vi "Autonomous Independent.vi"   [LabVIEW 2015]
doc: "This VI is called when autonomous begins, and will automatically be terminated when autonomous ends. You can carry out timed or sensor driven robot movement independently without needing to return to the caller."
uses:
  <vilib>/Rock Robotics/WPI/Utilities/WPI_GetSetVariantRefNum.vi
  <vilib>/Rock Robotics/Network Tables/NT Read Number.vi
  Robot Global Data.vi
  <vilib>/Rock Robotics/WPI/RobotDrive/WPI_RobotDriveMecanumDrive_Cartesian.vi
  <vilib>/Rock Robotics/Network Tables/NT Write Numeric Array.vi
panel:
  # "Be sure to right-click and choose Data Operations>>Make Current Value default if you want to save the array values with the VI"
types:
  T1 = typedef "WPI_JoystickDevRef.ctl" = cluster{"Device":T2}
  T2 = typedef "WPI_JoystickDeviceEnum.ctl" = enum16{"USB 0", "USB 1", "USB 2", "USB 3", "USB 4", "USB 5"}
  T3 = typedef "WPI_RobotDriveDevRef.ctl" = cluster{"DevStatus":errorcluster, "Motors[]":T4[], "Square Inputs":bool, "Max Output":dbl}
  T4 = typedef "WPI_MotorControlDeviceRef.ctl" = cluster{"DeviceStatus":errorcluster, "Type":T5, "PWM":cluster{"PWM Channel":T6, "DeadBand":T7}, "CAN":cluster{"Device Number":u8, "Control Mode":T8, "Semaphore":T9, "Max Vout":dbl, "TalonSRX Control Mode":T10}, "Invert":bool}
  T5 = typedef "WPI_MotorControlType.ctl" = enum16{"PWM", "CAN", "CANTalonSRX"}
  T6 = typedef "FPGA_DIOPWMChannel.ctl" = enum8{"PWM 0", "PWM 1", "PWM 2", "PWM 3", "PWM 4", "PWM 5", "PWM 6", "PWM 7", "PWM 8", "PWM 9", "PWM MXP 0", "PWM MXP 1", "PWM MXP 2", "PWM MXP 3", "PWM MXP 4", "PWM MXP 5", "PWM MXP 6", "PWM MXP 7", "PWM MXP 8", "PWM MXP 9", "Invalid"}
  T7 = typedef "WPI_PWMDeadband.ctl" = cluster{"Name":string, "maxPositivePwm":i32, "minPositivePwm":i32, "centerPwm":i32, "maxNegativePwm":i32, "minNegativePwm":i32, "angularRange":u16}
  T8 = typedef "WPI_CANJaguar_ControlMode.ctl" = enum8{"Percent VBus", "Current", "Speed", "Position", "Voltage"}
  T9 = typedef "Semaphore RefNum" = refnum<k1>
  T10 = typedef "WPI_CANTalonSRX_APIControlMode.ctl" = enum8{"Percent VBus", "Speed", "Position", "Slave", "Unchanged / Invalid", "Voltage Compensation", "Current", "Motion Profile"}
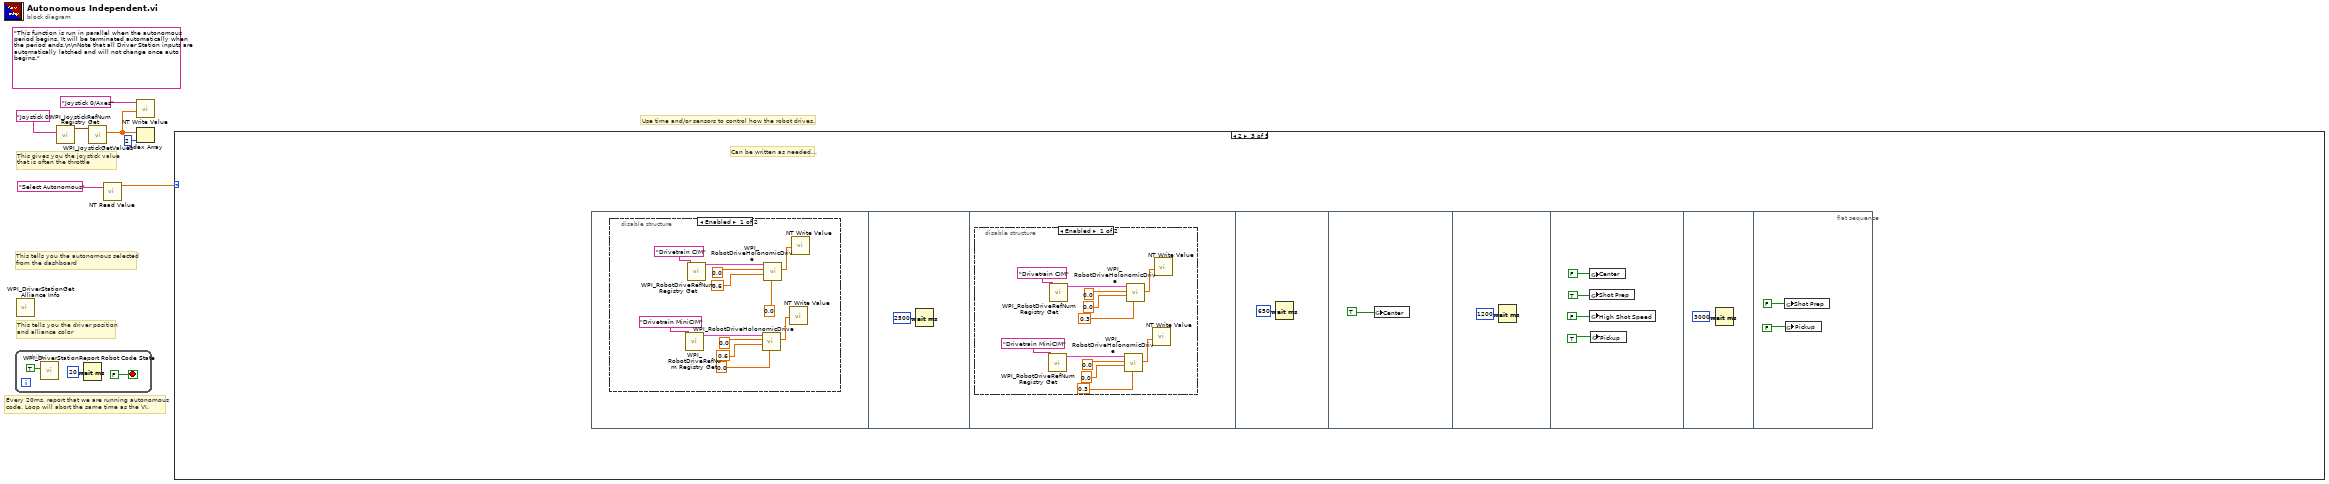
[diagram p0: block diagram]
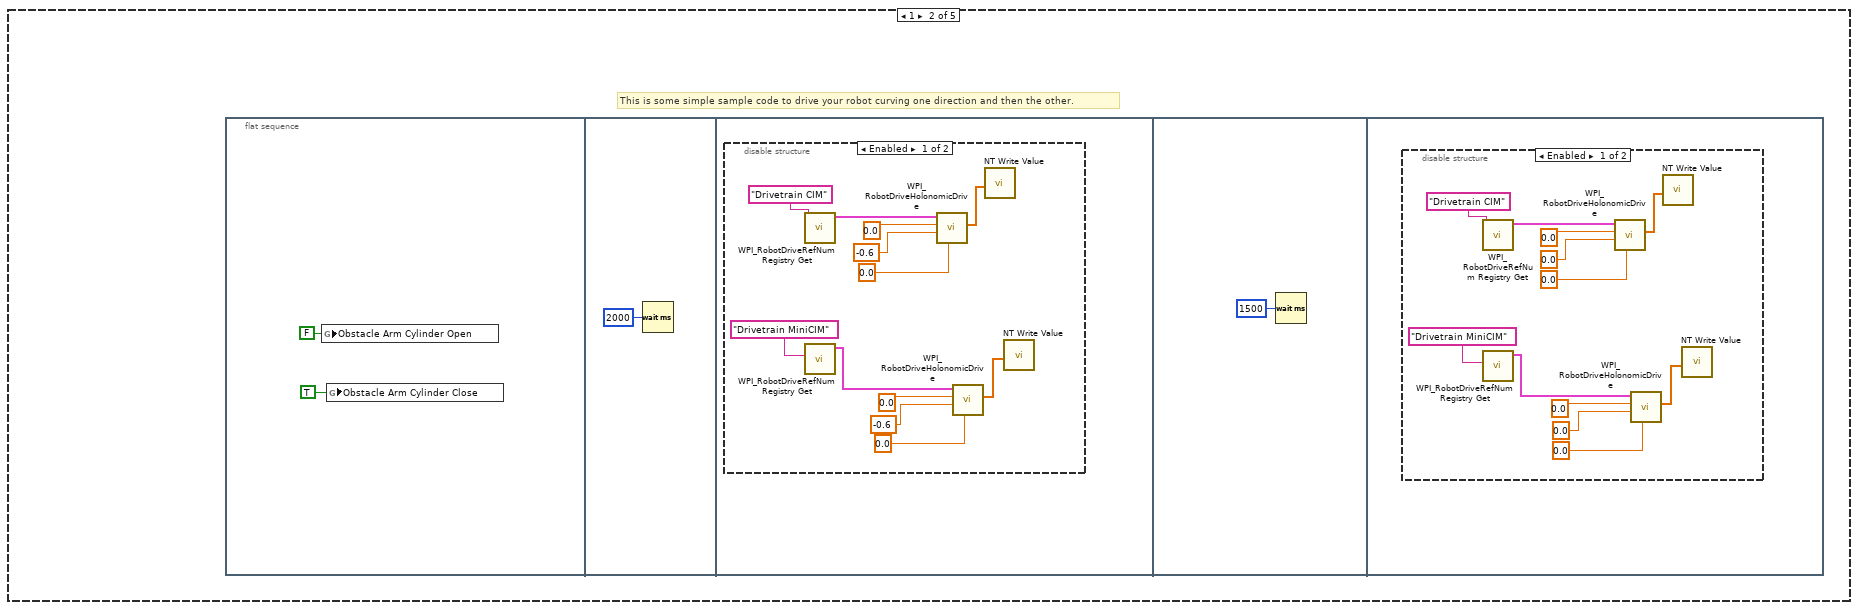
[diagram p3: hidden frame]
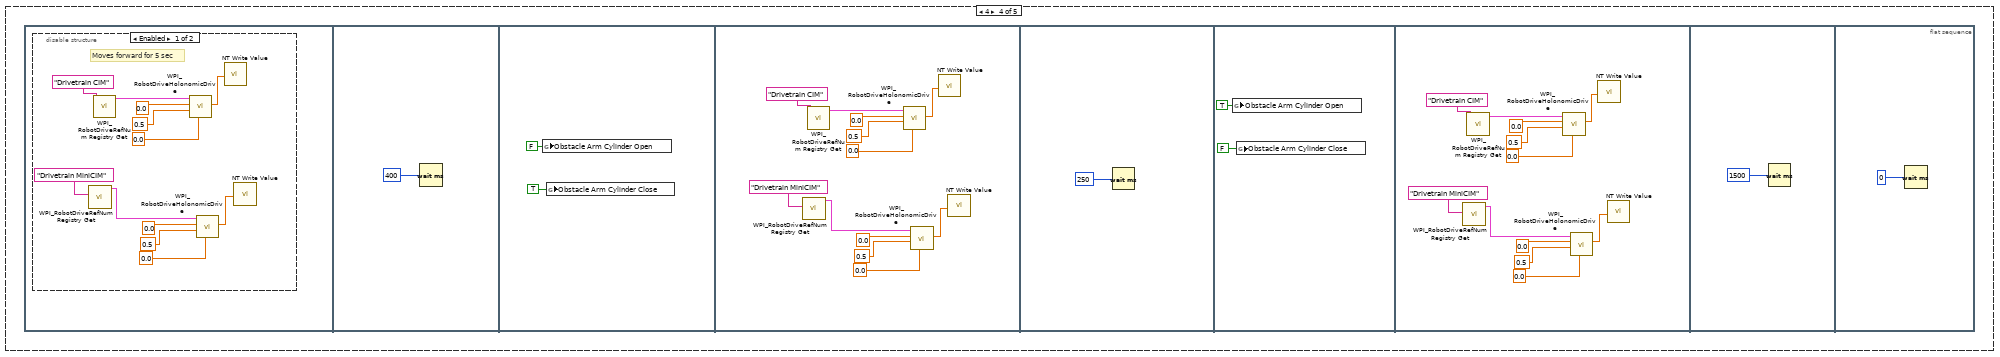
[diagram p8: hidden frame]
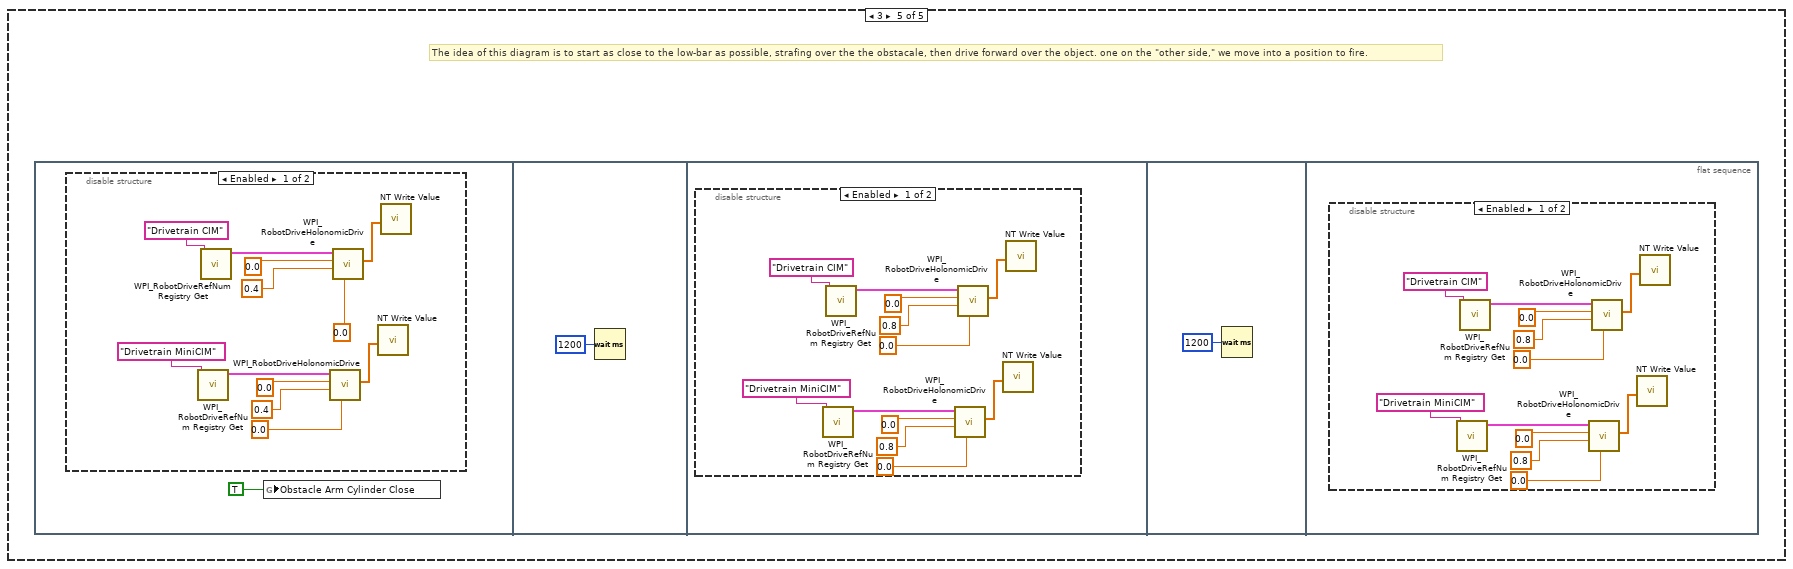
[diagram p10: hidden frame]
diagram:
  (unwired) "This function is run in parallel when the autonomous period begins. It will be terminated automatically when the period ends.\n\nNote that all Driver Station inputs are automatically latched and will not change once auto begins."
  # "This tells you the autonomous selected\nfrom the dashboard"
  # "Every 20ms, report that we are running autonomous\ncode. Loop will abort the same time as the VI."
  # "This gives you the joystick value\nthat is often the throttle"
  # "Use time and/or sensors to control how the robot drives."
  # "This tells you the driver position\nand alliance color"
  n1 = while {
    stop <- FALSE stop-if-true
    n2 = call <vilib>:"WPI_DriverStationReport Robot Code State.vi"("Autonomous"=TRUE) -> ()  [unwired: 10 in, 1 out]
    n3 = Wait (ms)(milliseconds to wait=u32 20) -> ()  [unwired: 1 out]
  }
  n4 = call <vilib>:"WPI_DriverStationGet Alliance Info.vi"() -> ()  [unwired: 12 out]
  n5 = call <vilib>:"WPI_JoystickRefNum Registry Get.vi"("refnum name"="Joystick 0") -> ("JoystickDevRef"=w6:T1)  [unwired: 1 in, 9 out]
  n6 = call <vilib>:"WPI_JoystickGetValues.vi"("JoystickDevRef"=w6) -> ("Axes"=w3:dbl[])  [unwired: 6 in, 4 out]
  n7 = call-poly <vilib>:"NT Read Value.vi"("Name"="Select Autonomous") -> ("Numeric"=w1:dbl)  [unwired: 9 in, 1 out]
  n8 = call-poly <vilib>:"NT Write Value.vi"("Numeric Array"=w3, "Name"="Joystick 0/Axes") -> ()  [unwired: 9 in, 1 out]
  n9 = Index Array(array=w3, index=2) -> ()  [unwired: 1 out]
  n10 = case shown="2" w1 {
    frame 0, Default {
    }
    frame 1 {
      # "This is some simple sample code to drive your robot curving one direction and then the other."
      n11 = flat-sequence {
        frame #0 {
          n12 = global write "Robot Global Data.vi" "Obstacle Arm Cylinder Open"(FALSE) -> ()
          n13 = global write "Robot Global Data.vi" "Obstacle Arm Cylinder Close"(TRUE) -> ()
        }
        frame #1 {
          n14 = Wait (ms)(milliseconds to wait=u32 2000) -> ()  [unwired: 1 out]
        }
        frame #2 {
          n15 = disable-structure shown="Enabled" {
            frame Enabled {
              n16 = call <vilib>:"WPI_RobotDriveRefNum Registry Get.vi"("refnum name"="Drivetrain CIM") -> ("RobotDriveDevRef"=w21:T3)  [unwired: 1 in, 9 out]
              n17 = call <vilib>:"WPI_RobotDriveRefNum Registry Get.vi"("refnum name"="Drivetrain MiniCIM") -> ("RobotDriveDevRef"=w15:T3)  [unwired: 1 in, 9 out]
              n18 = call-poly <vilib>:"WPI_RobotDriveHolonomicDrive.vi"("Rotation"=0.0, "Y"=-0.6 ("X axis value"), "X"=0.0 ("X axis value"), "RobotDriveDevRef"=w21) -> ("Motor Values"=w22:dbl[])  [unwired: 5 in, 2 out]
              n19 = call-poly <vilib>:"WPI_RobotDriveHolonomicDrive.vi"("Rotation"=0.0, "Y"=-0.6 ("X axis value"), "X"=0.0 ("X axis value"), "RobotDriveDevRef"=w15) -> ("Motor Values"=w17:dbl[])  [unwired: 5 in, 2 out]
              n20 = call-poly <vilib>:"NT Write Value.vi"("Numeric Array"=w22) -> ()  [unwired: 10 in, 1 out]
              n21 = call-poly <vilib>:"NT Write Value.vi"("Numeric Array"=w17) -> ()  [unwired: 10 in, 1 out]
            }
            frame Disabled {
            }
          }
        }
        frame #3 {
          n22 = Wait (ms)(milliseconds to wait=u32 1500) -> ()  [unwired: 1 out]
        }
        frame #4 {
          n23 = disable-structure shown="Enabled" {
            frame Enabled {
              n24 = call <vilib>:"WPI_RobotDriveRefNum Registry Get.vi"("refnum name"="Drivetrain CIM") -> ("RobotDriveDevRef"=w34:T3)  [unwired: 1 in, 9 out]
              n25 = call <vilib>:"WPI_RobotDriveRefNum Registry Get.vi"("refnum name"="Drivetrain MiniCIM") -> ("RobotDriveDevRef"=w28:T3)  [unwired: 1 in, 9 out]
              n26 = call-poly <vilib>:"WPI_RobotDriveHolonomicDrive.vi"("Rotation"=0.0, "Y"=0.0 ("X axis value"), "X"=0.0 ("X axis value"), "RobotDriveDevRef"=w34) -> ("Motor Values"=w35:dbl[])  [unwired: 5 in, 2 out]
              n27 = call-poly <vilib>:"WPI_RobotDriveHolonomicDrive.vi"("Rotation"=0.0, "Y"=0.0 ("X axis value"), "X"=0.0 ("X axis value"), "RobotDriveDevRef"=w28) -> ("Motor Values"=w30:dbl[])  [unwired: 5 in, 2 out]
              n28 = call-poly <vilib>:"NT Write Value.vi"("Numeric Array"=w35) -> ()  [unwired: 10 in, 1 out]
              n29 = call-poly <vilib>:"NT Write Value.vi"("Numeric Array"=w30) -> ()  [unwired: 10 in, 1 out]
            }
            frame Disabled {
            }
          }
        }
      }
    }
    frame 2 {
      # "Can be written as needed..."
      n30 = flat-sequence {
        frame #0 {
          n31 = disable-structure shown="Enabled" {
            frame Enabled {
              n32 = call <vilib>:"WPI_RobotDriveRefNum Registry Get.vi"("refnum name"="Drivetrain MiniCIM") -> ("RobotDriveDevRef"=w40:T3)  [unwired: 1 in, 9 out]
              n33 = call <vilib>:"WPI_RobotDriveRefNum Registry Get.vi"("refnum name"="Drivetrain CIM") -> ("RobotDriveDevRef"=w46:T3)  [unwired: 1 in, 9 out]
              n34 = call-poly <vilib>:"WPI_RobotDriveHolonomicDrive.vi"("Rotation"=0.0, "Y"=0.6 ("X axis value"), "X"=0.0 ("X axis value"), "RobotDriveDevRef"=w40) -> ("Motor Values"=w41:dbl[])  [unwired: 5 in, 2 out]
              n35 = call-poly <vilib>:"WPI_RobotDriveHolonomicDrive.vi"("Rotation"=0.0, "Y"=0.6 ("X axis value"), "X"=0.0 ("X axis value"), "RobotDriveDevRef"=w46) -> ("Motor Values"=w47:dbl[])  [unwired: 5 in, 2 out]
              n36 = call-poly <vilib>:"NT Write Value.vi"("Numeric Array"=w41) -> ()  [unwired: 10 in, 1 out]
              n37 = call-poly <vilib>:"NT Write Value.vi"("Numeric Array"=w47) -> ()  [unwired: 10 in, 1 out]
            }
            frame Disabled {
            }
          }
        }
        frame #1 {
          n38 = Wait (ms)(milliseconds to wait=u32 2500) -> ()  [unwired: 1 out]
        }
        frame #2 {
          n39 = disable-structure shown="Enabled" {
            frame Enabled {
              n40 = call <vilib>:"WPI_RobotDriveRefNum Registry Get.vi"("refnum name"="Drivetrain MiniCIM") -> ("RobotDriveDevRef"=w53:T3)  [unwired: 1 in, 9 out]
              n41 = call <vilib>:"WPI_RobotDriveRefNum Registry Get.vi"("refnum name"="Drivetrain CIM") -> ("RobotDriveDevRef"=w59:T3)  [unwired: 1 in, 9 out]
              n42 = call-poly <vilib>:"WPI_RobotDriveHolonomicDrive.vi"("Rotation"=0.3, "Y"=0.0 ("X axis value"), "X"=0.0 ("X axis value"), "RobotDriveDevRef"=w53) -> ("Motor Values"=w54:dbl[])  [unwired: 5 in, 2 out]
              n43 = call-poly <vilib>:"WPI_RobotDriveHolonomicDrive.vi"("Rotation"=0.3, "Y"=0.0 ("X axis value"), "X"=0.0 ("X axis value"), "RobotDriveDevRef"=w59) -> ("Motor Values"=w60:dbl[])  [unwired: 5 in, 2 out]
              n44 = call-poly <vilib>:"NT Write Value.vi"("Numeric Array"=w54) -> ()  [unwired: 10 in, 1 out]
              n45 = call-poly <vilib>:"NT Write Value.vi"("Numeric Array"=w60) -> ()  [unwired: 10 in, 1 out]
            }
            frame Disabled {
            }
          }
        }
        frame #3 {
          n46 = Wait (ms)(milliseconds to wait=u32 650) -> ()  [unwired: 1 out]
        }
        frame #4 {
          n47 = global write "Robot Global Data.vi" "Center"(TRUE) -> ()
        }
        frame #5 {
          n48 = Wait (ms)(milliseconds to wait=u32 1200) -> ()  [unwired: 1 out]
        }
        frame #6 {
          n49 = global write "Robot Global Data.vi" "Center"(FALSE) -> ()
          n50 = global write "Robot Global Data.vi" "Shot Prep"(TRUE) -> ()
          n51 = global write "Robot Global Data.vi" "High Shot Speed"(FALSE) -> ()
          n52 = global write "Robot Global Data.vi" "Pickup"(TRUE) -> ()
        }
        frame #7 {
          n53 = Wait (ms)(milliseconds to wait=u32 3000) -> ()  [unwired: 1 out]
        }
        frame #8 {
          n54 = global write "Robot Global Data.vi" "Shot Prep"(FALSE) -> ()
          n55 = global write "Robot Global Data.vi" "Pickup"(FALSE) -> ()
        }
      }
    }
    frame 4 {
      n56 = flat-sequence {
        frame #0 {
          n57 = disable-structure shown="Enabled" {
            frame Enabled {
              # "Moves forward for 5 sec"
              n58 = call <vilib>:"WPI_RobotDriveRefNum Registry Get.vi"("refnum name"="Drivetrain MiniCIM") -> ("RobotDriveDevRef"=w75:T3)  [unwired: 1 in, 9 out]
              n59 = call <vilib>:"WPI_RobotDriveRefNum Registry Get.vi"("refnum name"="Drivetrain CIM") -> ("RobotDriveDevRef"=w81:T3)  [unwired: 1 in, 9 out]
              n60 = call-poly <vilib>:"WPI_RobotDriveHolonomicDrive.vi"("Rotation"=0.0, "Y"=0.5 ("X axis value"), "X"=0.0 ("X axis value"), "RobotDriveDevRef"=w81) -> ("Motor Values"=w82:dbl[])  [unwired: 5 in, 2 out]
              n61 = call-poly <vilib>:"WPI_RobotDriveHolonomicDrive.vi"("Rotation"=0.0, "Y"=0.5 ("X axis value"), "X"=0.0 ("X axis value"), "RobotDriveDevRef"=w75) -> ("Motor Values"=w77:dbl[])  [unwired: 5 in, 2 out]
              n62 = call-poly <vilib>:"NT Write Value.vi"("Numeric Array"=w82) -> ()  [unwired: 10 in, 1 out]
              n63 = call-poly <vilib>:"NT Write Value.vi"("Numeric Array"=w77) -> ()  [unwired: 10 in, 1 out]
            }
            frame Disabled {
            }
          }
        }
        frame #1 {
          n64 = Wait (ms)(milliseconds to wait=u32 400) -> ()  [unwired: 1 out]
        }
        frame #2 {
          n65 = global write "Robot Global Data.vi" "Obstacle Arm Cylinder Open"(FALSE) -> ()
          n66 = global write "Robot Global Data.vi" "Obstacle Arm Cylinder Close"(TRUE) -> ()
        }
        frame #3 {
          n67 = call <vilib>:"WPI_RobotDriveRefNum Registry Get.vi"("refnum name"="Drivetrain MiniCIM") -> ("RobotDriveDevRef"=w90:T3)  [unwired: 1 in, 9 out]
          n68 = call <vilib>:"WPI_RobotDriveRefNum Registry Get.vi"("refnum name"="Drivetrain CIM") -> ("RobotDriveDevRef"=w96:T3)  [unwired: 1 in, 9 out]
          n69 = call-poly <vilib>:"WPI_RobotDriveHolonomicDrive.vi"("Rotation"=0.0, "Y"=0.5 ("X axis value"), "X"=0.0 ("X axis value"), "RobotDriveDevRef"=w96) -> ("Motor Values"=w97:dbl[])  [unwired: 5 in, 2 out]
          n70 = call-poly <vilib>:"WPI_RobotDriveHolonomicDrive.vi"("Rotation"=0.0, "Y"=0.5 ("X axis value"), "X"=0.0 ("X axis value"), "RobotDriveDevRef"=w90) -> ("Motor Values"=w92:dbl[])  [unwired: 5 in, 2 out]
          n71 = call-poly <vilib>:"NT Write Value.vi"("Numeric Array"=w97) -> ()  [unwired: 10 in, 1 out]
          n72 = call-poly <vilib>:"NT Write Value.vi"("Numeric Array"=w92) -> ()  [unwired: 10 in, 1 out]
        }
        frame #4 {
          n73 = Wait (ms)(milliseconds to wait=u32 250) -> ()  [unwired: 1 out]
        }
        frame #5 {
          n74 = global write "Robot Global Data.vi" "Obstacle Arm Cylinder Open"(TRUE) -> ()
          n75 = global write "Robot Global Data.vi" "Obstacle Arm Cylinder Close"(FALSE) -> ()
        }
        frame #6 {
          n76 = call <vilib>:"WPI_RobotDriveRefNum Registry Get.vi"("refnum name"="Drivetrain MiniCIM") -> ("RobotDriveDevRef"=w105:T3)  [unwired: 1 in, 9 out]
          n77 = call <vilib>:"WPI_RobotDriveRefNum Registry Get.vi"("refnum name"="Drivetrain CIM") -> ("RobotDriveDevRef"=w111:T3)  [unwired: 1 in, 9 out]
          n78 = call-poly <vilib>:"WPI_RobotDriveHolonomicDrive.vi"("Rotation"=0.0, "Y"=0.5 ("X axis value"), "X"=0.0 ("X axis value"), "RobotDriveDevRef"=w111) -> ("Motor Values"=w112:dbl[])  [unwired: 5 in, 2 out]
          n79 = call-poly <vilib>:"WPI_RobotDriveHolonomicDrive.vi"("Rotation"=0.0, "Y"=0.5 ("X axis value"), "X"=0.0 ("X axis value"), "RobotDriveDevRef"=w105) -> ("Motor Values"=w107:dbl[])  [unwired: 5 in, 2 out]
          n80 = call-poly <vilib>:"NT Write Value.vi"("Numeric Array"=w112) -> ()  [unwired: 10 in, 1 out]
          n81 = call-poly <vilib>:"NT Write Value.vi"("Numeric Array"=w107) -> ()  [unwired: 10 in, 1 out]
        }
        frame #7 {
          n82 = Wait (ms)(milliseconds to wait=u32 1500) -> ()  [unwired: 1 out]
        }
        frame #8 {
          n83 = Wait (ms)(milliseconds to wait=u32 0) -> ()  [unwired: 1 out]
        }
      }
    }
    frame 3 {
      # "The idea of this diagram is to start as close to the low-bar as possible, strafing over the the obstacale, then drive forward over the object. one on the \"other side,\" we move into a position to fire."
      n84 = flat-sequence {
        frame #0 {
          n85 = disable-structure shown="Enabled" {
            frame Enabled {
              n86 = call <vilib>:"WPI_RobotDriveRefNum Registry Get.vi"("refnum name"="Drivetrain MiniCIM") -> ("RobotDriveDevRef"=w120:T3)  [unwired: 1 in, 9 out]
              n87 = call <vilib>:"WPI_RobotDriveRefNum Registry Get.vi"("refnum name"="Drivetrain CIM") -> ("RobotDriveDevRef"=w126:T3)  [unwired: 1 in, 9 out]
              n88 = call-poly <vilib>:"WPI_RobotDriveHolonomicDrive.vi"("Rotation"=0.0, "Y"=0.4 ("X axis value"), "X"=0.0 ("X axis value"), "RobotDriveDevRef"=w120) -> ("Motor Values"=w121:dbl[])  [unwired: 5 in, 2 out]
              n89 = call-poly <vilib>:"WPI_RobotDriveHolonomicDrive.vi"("Rotation"=0.0, "Y"=0.4 ("X axis value"), "X"=0.0 ("X axis value"), "RobotDriveDevRef"=w126) -> ("Motor Values"=w127:dbl[])  [unwired: 5 in, 2 out]
              n90 = call-poly <vilib>:"NT Write Value.vi"("Numeric Array"=w121) -> ()  [unwired: 10 in, 1 out]
              n91 = call-poly <vilib>:"NT Write Value.vi"("Numeric Array"=w127) -> ()  [unwired: 10 in, 1 out]
            }
            frame Disabled {
            }
          }
          n92 = global write "Robot Global Data.vi" "Obstacle Arm Cylinder Close"(TRUE) -> ()
        }
        frame #1 {
          n93 = Wait (ms)(milliseconds to wait=u32 1200) -> ()  [unwired: 1 out]
        }
        frame #2 {
          n94 = disable-structure shown="Enabled" {
            frame Enabled {
              n95 = call <vilib>:"WPI_RobotDriveRefNum Registry Get.vi"("refnum name"="Drivetrain MiniCIM") -> ("RobotDriveDevRef"=w133:T3)  [unwired: 1 in, 9 out]
              n96 = call <vilib>:"WPI_RobotDriveRefNum Registry Get.vi"("refnum name"="Drivetrain CIM") -> ("RobotDriveDevRef"=w139:T3)  [unwired: 1 in, 9 out]
              n97 = call-poly <vilib>:"WPI_RobotDriveHolonomicDrive.vi"("Rotation"=0.0, "Y"=0.8 ("X axis value"), "X"=0.0 ("X axis value"), "RobotDriveDevRef"=w133) -> ("Motor Values"=w134:dbl[])  [unwired: 5 in, 2 out]
              n98 = call-poly <vilib>:"WPI_RobotDriveHolonomicDrive.vi"("Rotation"=0.0, "Y"=0.8 ("X axis value"), "X"=0.0 ("X axis value"), "RobotDriveDevRef"=w139) -> ("Motor Values"=w140:dbl[])  [unwired: 5 in, 2 out]
              n99 = call-poly <vilib>:"NT Write Value.vi"("Numeric Array"=w134) -> ()  [unwired: 10 in, 1 out]
              n100 = call-poly <vilib>:"NT Write Value.vi"("Numeric Array"=w140) -> ()  [unwired: 10 in, 1 out]
            }
            frame Disabled {
            }
          }
        }
        frame #3 {
          n101 = Wait (ms)(milliseconds to wait=u32 1200) -> ()  [unwired: 1 out]
        }
        frame #4 {
          n102 = disable-structure shown="Enabled" {
            frame Enabled {
              n103 = call <vilib>:"WPI_RobotDriveRefNum Registry Get.vi"("refnum name"="Drivetrain MiniCIM") -> ("RobotDriveDevRef"=w146:T3)  [unwired: 1 in, 9 out]
              n104 = call <vilib>:"WPI_RobotDriveRefNum Registry Get.vi"("refnum name"="Drivetrain CIM") -> ("RobotDriveDevRef"=w152:T3)  [unwired: 1 in, 9 out]
              n105 = call-poly <vilib>:"WPI_RobotDriveHolonomicDrive.vi"("Rotation"=0.0, "Y"=0.8 ("X axis value"), "X"=0.0 ("X axis value"), "RobotDriveDevRef"=w146) -> ("Motor Values"=w147:dbl[])  [unwired: 5 in, 2 out]
              n106 = call-poly <vilib>:"WPI_RobotDriveHolonomicDrive.vi"("Rotation"=0.0, "Y"=0.8 ("X axis value"), "X"=0.0 ("X axis value"), "RobotDriveDevRef"=w152) -> ("Motor Values"=w153:dbl[])  [unwired: 5 in, 2 out]
              n107 = call-poly <vilib>:"NT Write Value.vi"("Numeric Array"=w147) -> ()  [unwired: 10 in, 1 out]
              n108 = call-poly <vilib>:"NT Write Value.vi"("Numeric Array"=w153) -> ()  [unwired: 10 in, 1 out]
            }
            frame Disabled {
            }
          }
        }
      }
    }
  }
